vi "CreateWorldAndBody.vi"(8 "error in (no error)":errorcluster, 11 "Snake in":refnum<class "Snake.lvclass">) -> (0 "error out":errorcluster, 3 "Snake out":refnum<class "Snake.lvclass">)   [LabVIEW 2014, in "Snake.lvclass"]
uses:
  Snake.lvclass
  Snake.lvclass/Snake.ctl
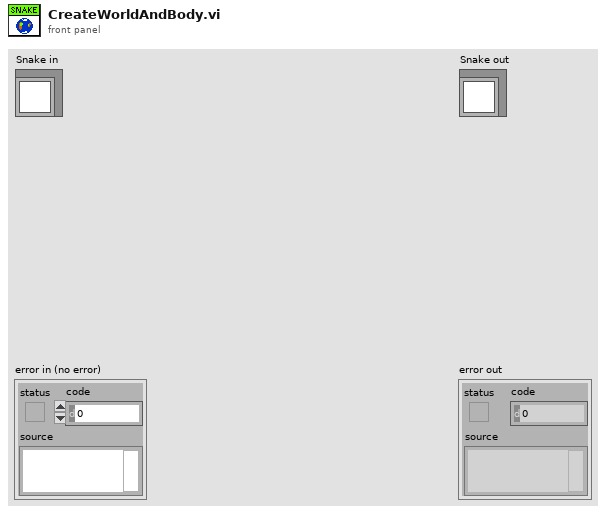
[diagram p1: front panel]
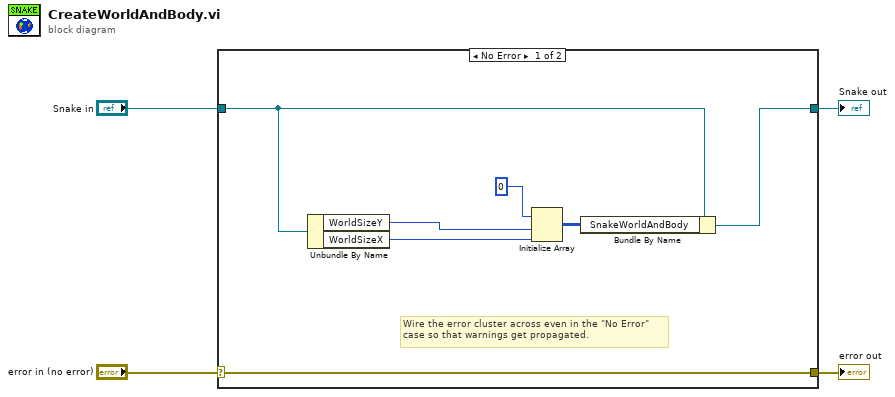
[diagram p0: block diagram]
diagram:
  n1 = case shown="No Error" "error in (no error)" {
    selector: "error in (no error)" -> [w11 w13]
    tunnel: [w11 w13] -> w3
    tunnel: [w9 w12] -> w1
    tunnel: "Snake in" -> [w7 w12]
    frame No Error {
      # "Wire the error cluster across even in the \"No Error\"\ncase so that warnings get propagated."
      n2 = Unbundle By Name(w7) -> ("WorldSizeY"=w6:i32, "WorldSizeX"=w5:i32)
      n3 = Initialize Array(u32 0, w6, w5) -> (w8:u32[][])
      n4 = Bundle By Name(cluster=w7, "SnakeWorldAndBody"=w8) -> (w9:refnum<class "Snake.lvclass">)
    }
    frame Error {
    }
  }
  "error out" <- w3
  "Snake out" <- w1
